vi "Serial_Dcoder.vi"(8 "RX Count":u32, 11 "string":string) -> (0 "StepForce":u8[](array[numeric]), 3 "OK":bool)   [LabVIEW 2017]
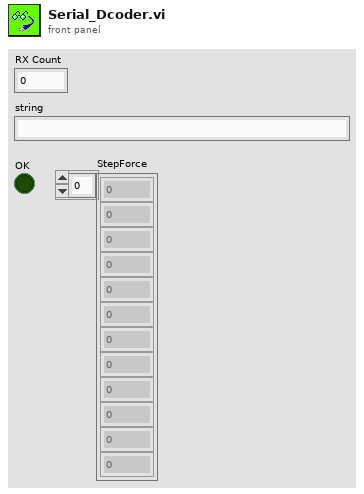
[diagram p1: front panel]
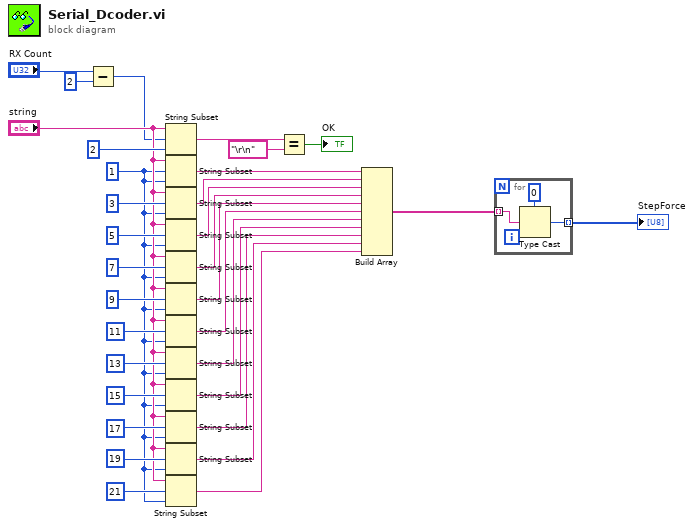
[diagram p0: block diagram]
diagram:
  w5 = 1 ("offset (0)")
  n1 = Subtract(x="RX Count", y=u32 2) -> (x-y=w1:u32)
  n2 = String Subset(string="string", offset (0)=w1, length (rest)=2 ("length (rest)")) -> (substring=w31:string)
  n3 = String Subset(string="string", offset (0)=w5, length (rest)=w5) -> (substring=w19:string)
  n4 = String Subset(string="string", offset (0)=3, length (rest)=w5) -> (substring=w18:string)
  n5 = String Subset(string="string", offset (0)=5, length (rest)=w5) -> (substring=w17:string)
  n6 = String Subset(string="string", offset (0)=7, length (rest)=w5) -> (substring=w16:string)
  n7 = String Subset(string="string", offset (0)=9, length (rest)=w5) -> (substring=w15:string)
  n8 = String Subset(string="string", offset (0)=11, length (rest)=w5) -> (substring=w14:string)
  n9 = String Subset(string="string", offset (0)=13, length (rest)=w5) -> (substring=w13:string)
  n10 = String Subset(string="string", offset (0)=15, length (rest)=w5) -> (substring=w12:string)
  n11 = String Subset(string="string", offset (0)=17, length (rest)=w5) -> (substring=w11:string)
  n12 = String Subset(string="string", offset (0)=19, length (rest)=w5) -> (substring=w10:string)
  n13 = String Subset(string="string", offset (0)=21, length (rest)=w5) -> (substring=w4:string)
  n14 = Equal?(x=w31, y="\r\n") -> (x = y?=→"OK":bool)
  n15 = Build Array(w19, w18, w17, w16, w15, w14, w13, w12, w11, w10, w4) -> (w9:string[])
  n16 = for {
    tunnel: w9 -> [w34] mode=indexing
    tunnel: [w33] -> w8 mode=indexing
    n17 = Type Cast(type=u8 0, x=w34) -> (*(type *) &x=w33:u8)
  }
  "StepForce" <- w8
